vi "origin_curve_fitting.vi"() -> ()   [LabVIEW 2014]
uses:
  <vilib>/Utility/file.llb/Read From Spreadsheet File (DBL).vi
panel:
  in  "generic data":bool
  in  "Fitting":bool
  in  "stop":bool
  in  "Fitting Function":string(combo)="lorentz"
  out "Peak Center":dbl
  out "Peak Width":dbl
  out "Adj. R-Square":dbl
  out "Fit":cluster{"data":dbl[], "data":dbl[]}[](graph)
  out "Origin ogw Load":bool
  out "ogw path":path
  out "data filepath":path
  in  "Visible":i32(ring) caption="Origin Visible" items=["MAINWND_HIDE"=0, "MAINWND_SHOW"=1, "MAINWND_SHOWMINIMIZED"=2, "MAINWND_SHOWMAXIMIZED"=3, "MAINWND_SHOW_BRING_TO_FRONT"=100]
  out "SettingsWks":refnum<k7>
  out "Input Data":cluster{"data":dbl[], "data":dbl[]}(graph)
  out "DataWks":refnum<k7>
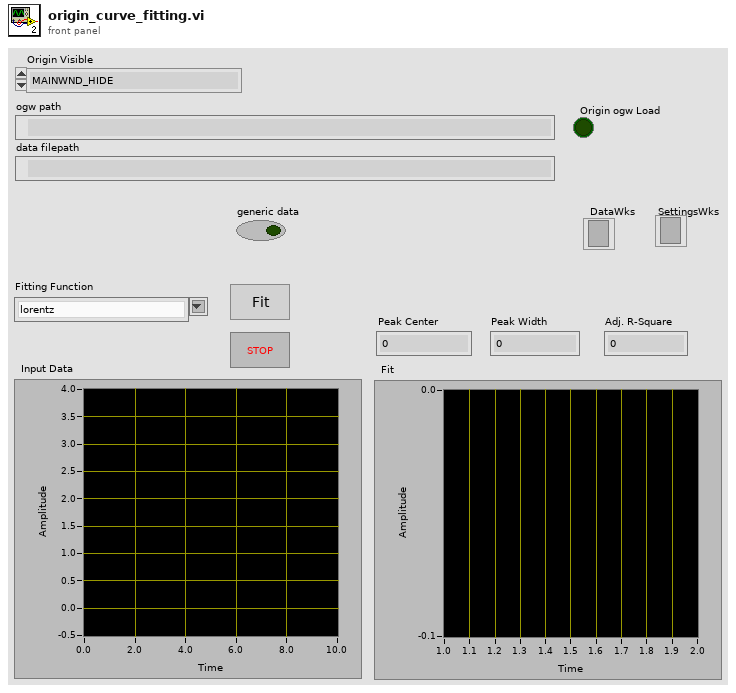
[diagram p1: front panel]
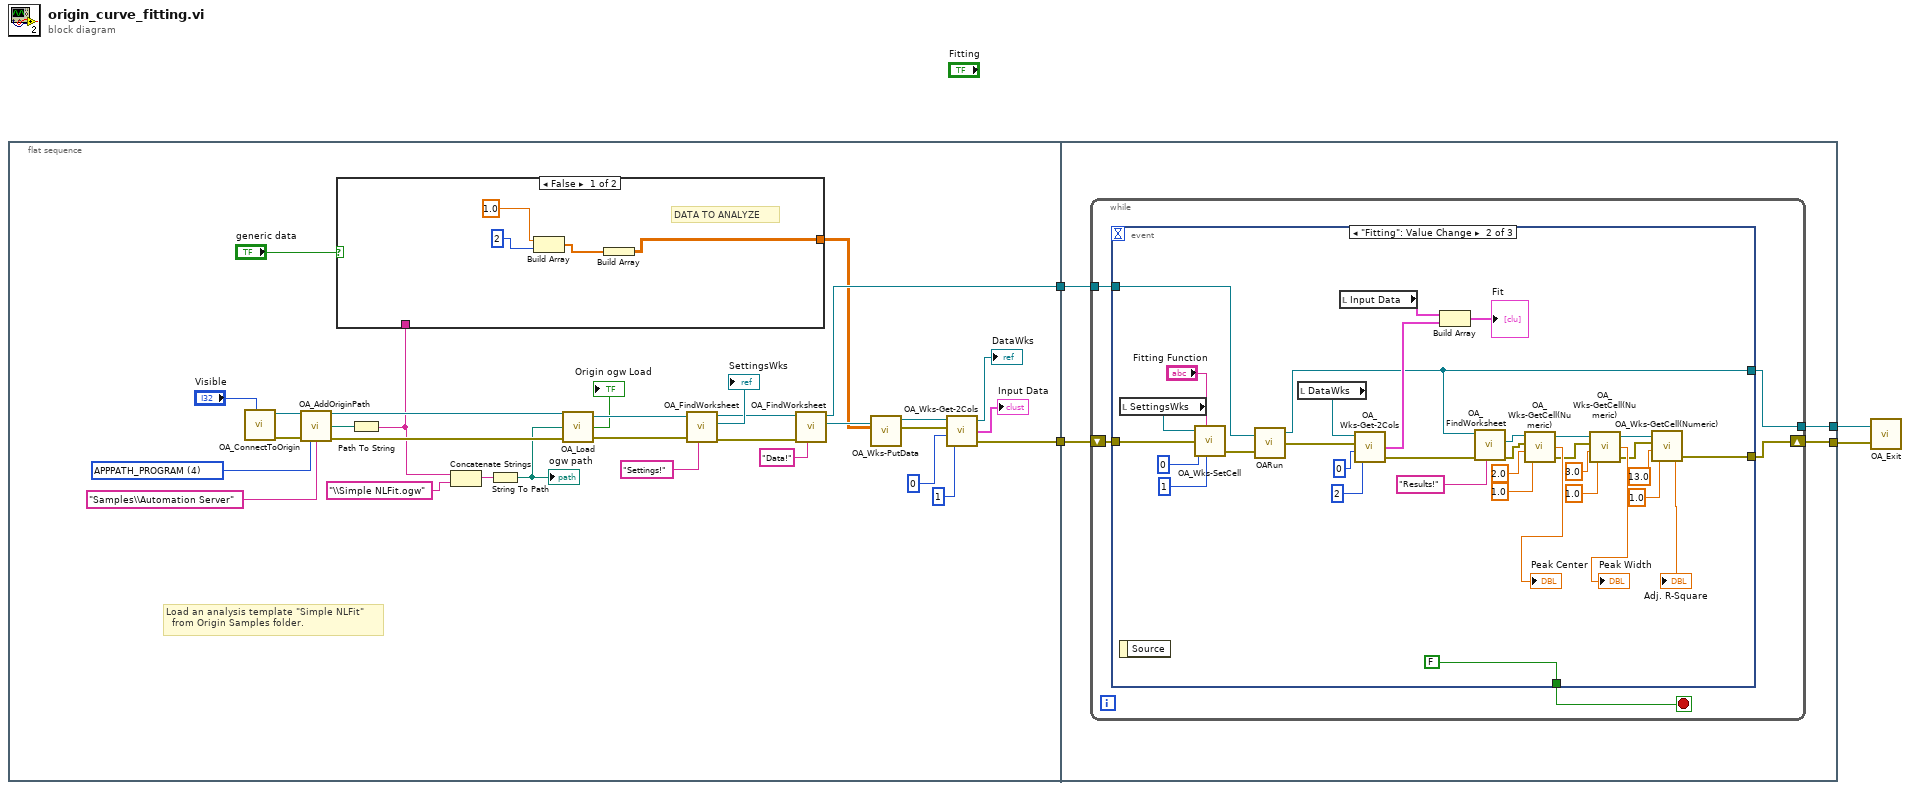
[diagram p0: block diagram]
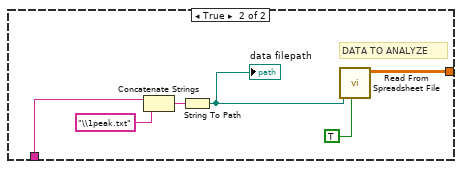
[diagram p2: hidden frame]
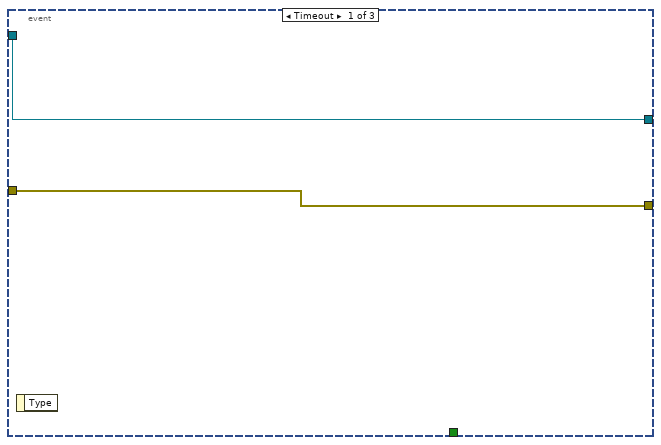
[diagram p3: hidden frame]
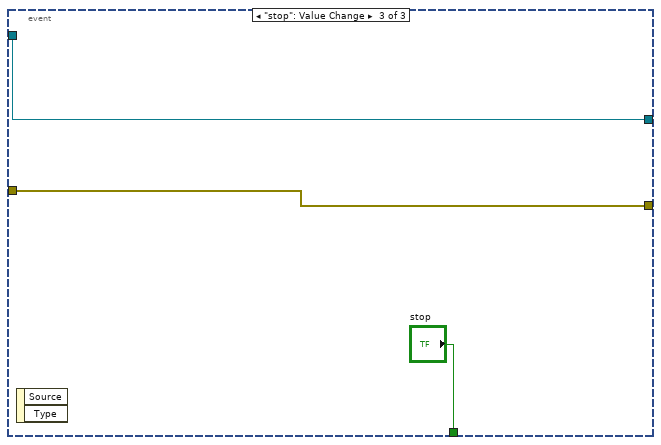
[diagram p4: hidden frame]
diagram:
  n1 = flat-sequence {
    tunnel: [w16] -> w4
    tunnel: [w12] -> w3
    tunnel: w4 -> [w49]
    tunnel: [w48] -> w2
    tunnel: w3 -> [w47]
    tunnel: [w46] -> w1
    frame #0 {
      w33 = 4 items=["APPPATH_USER"=2, "APPPATH_GROUP"=3, "APPPATH_PROGRAM"=4] ("Type")
      # "Load an analysis template \"Simple NLFit\"\n  from Origin Samples folder."
      n2 = call <userlib>:"OA_ConnectToOrigin.vi"("Visible"="Visible") -> ("error out"=w28:errorcluster, "Origin.IOApplication"=w29:refnum<k7>)  [unwired: 7 in]
      n3 = call <userlib>:"OA_AddOriginPath.vi"("Origin.IOApplication"=w29, "error in (no error)"=w28, "Type"=w33, "Filename"="Samples\\Automation Server") -> ("Origin.IOApplication"=w35:refnum<k7>, "path out"=w23:path, "error out"=w34:errorcluster)  [unwired: 9 in]
      n4 = Path To String(path=w23) -> (string=w6:string)
      n5 = case shown="False" "generic data" {
        tunnel: [w36 w41] -> w7
        tunnel: w6 -> [_ w40]
        frame False {
          # "DATA TO ANALYZE"
          n6 = Build Array(1.0, 2) -> (w37:dbl[])
          n7 = Build Array(w37) -> (w36:dbl[][])
        }
        frame True {
          # "DATA TO ANALYZE"
          n8 = Concatenate Strings(w40, "\\1peak.txt" ("string")) -> (w45:string)
          n9 = String To Path(string=w45) -> (path=w42:path)
          "data filepath" <- w42
          n10 = call-poly <vilib>:"Read From Spreadsheet File.vi"("transpose (no:F)"=TRUE, "file path (dialog if empty)"=w42) -> ("all rows"=w41:dbl[][])  [unwired: 5 in, 4 out]
        }
      }
      n11 = Concatenate Strings(w6, "\\Simple NLFit.ogw" ("string")) -> (w25:string)
      n12 = String To Path(string=w25) -> (path=w24:path)
      "ogw path" <- w24
      n13 = call <userlib>:"OA_Load.vi"("error in (no error)"=w34, "Path"=w24, "Origin.IOApplication"=w35) -> ("error out"=w30:errorcluster, "Load"=→"Origin ogw Load":bool, "Origin.IOApplication"=w31:refnum<k7>)
      n14 = call <userlib>:"OA_FindWorksheet.vi"("Name"="Settings!", "error in (no error)"=w30, "Origin.IOApplication"=w31) -> ("error out"=w17:errorcluster, "Origin.Worksheet"=→"SettingsWks":refnum<k7>, "Origin.IOApplication"=w19:refnum<k7>)  [unwired: 6 in]
      n15 = call <userlib>:"OA_FindWorksheet.vi"("Name"="Data!", "error in (no error)"=w17, "Origin.IOApplication"=w19) -> ("Origin.Worksheet"=w11:refnum<k7>, "Origin.IOApplication"=w12:refnum<k7>)  [unwired: 6 in, 1 out]
      n16 = call <userlib>:"OA_Wks-PutData.vi"("2d Data"=w7, "Origin.Worksheet"=w11) -> ("error out"=w9:errorcluster, "Origin.Worksheet Out"=w10:refnum<k7>)  [unwired: 3 in, 1 out]
      n17 = call <userlib>:"OA_Wks-Get-2Cols.vi"("yCol"=1, "xCol"=0, "error in (no error)"=w9, "Origin.Worksheet"=w10) -> ("error out"=w16:errorcluster, "Bundled Cols"=→"Input Data":cluster{"data":dbl[], "data":dbl[]}, "Origin.Worksheet Dup"=→"DataWks":refnum<k7>)
    }
    frame #1 {
      n18 = while {
        shift-right: [w53] -> w48
        shift-left: w49 -> [w54]
        tunnel: w47 -> [w51]
        tunnel: [w50] -> w46
        stop <- w52 stop-if-true
        n19 = event shown="[1] \"Fitting\": Value Change" {
          selector: _ -> [_ _ _]
          dyn-events: _ -> [_ _ _]
          timeout: _ -> [_ _ _]
          tunnel: w54 -> [w56 w67 w92]
          tunnel: [w56 w57 w92] -> w53
          tunnel: [_ FALSE "stop"] -> w52
          tunnel: w51 -> [w55 w64 w91]
          tunnel: [w55 w58 w91] -> w50
          event Timeout {
            n20 = event-data() -> ()  [unwired: 1 in, 1 out]
          }
          event "Fitting": Value Change {
            n21 = local read "SettingsWks"() -> (w87:refnum<k7>)
            n22 = event-data() -> ()  [unwired: 1 in, 1 out]
            n23 = call <userlib>:"OA_Wks-SetCell.vi"("Origin.Worksheet"=w87, "Data"="Fitting Function", "error in (no error)"=w67, "r1"=0, "c1"=1) -> ("error out"=w60:errorcluster)  [unwired: 2 out]
            n24 = call <userlib>:"OARun.vi"("Origin.IOApplication"=w64, "Error IO"=w60) -> ("Origin.IOApplication"=w58:refnum<k7>, "Error IO Out"=w66:errorcluster)  [unwired: 1 out]
            n25 = local read "DataWks"() -> (w59:refnum<k7>)
            n26 = local read "Input Data"() -> (w62:cluster{"data":dbl[], "data":dbl[]})
            n27 = call <userlib>:"OA_Wks-Get-2Cols.vi"("yCol"=2, "xCol"=0, "error in (no error)"=w66, "Origin.Worksheet"=w59) -> ("error out"=w68:errorcluster, "Bundled Cols"=w63:cluster{"data":dbl[], "data":dbl[]})  [unwired: 1 out]
            n28 = Build Array(w62, w63) -> (→"Fit":cluster{"data":dbl[], "data":dbl[]}[])
            n29 = call <userlib>:"OA_FindWorksheet.vi"("Name"="Results!", "error in (no error)"=w68, "Origin.IOApplication"=w58) -> ("error out"=w84:errorcluster, "Origin.Worksheet"=w85:refnum<k7>)  [unwired: 6 in, 1 out]
            n30 = call <userlib>:"OA_Wks-GetCell(Numeric).vi"("c1"=1.0, "r1"=2.0, "error in (no error)"=w84, "Origin.Worksheet"=w85) -> ("error out"=w79:errorcluster, "Data"=→"Peak Center":dbl, "Origin.Worksheet Out"=w80:refnum<k7>)
            n31 = call <userlib>:"OA_Wks-GetCell(Numeric).vi"("c1"=1.0, "r1"=3.0, "error in (no error)"=w79, "Origin.Worksheet"=w80) -> ("error out"=w74:errorcluster, "Data"=→"Peak Width":dbl, "Origin.Worksheet Out"=w75:refnum<k7>)
            n32 = call <userlib>:"OA_Wks-GetCell(Numeric).vi"("c1"=1.0, "r1"=13.0, "error in (no error)"=w74, "Origin.Worksheet"=w75) -> ("error out"=w57:errorcluster, "Data"=→"Adj. R-Square":dbl)  [unwired: 1 out]
          }
          event "stop": Value Change {
            n33 = event-data() -> ()  [unwired: 1 in, 2 out]
          }
        }
      }
    }
  }
  n34 = call <userlib>:"OA_Exit.vi"("Error IO"=w2, "Origin.IOApplication"=w1) -> ()  [unwired: 2 out]
